vi "PH_Switch.calc State.vi"(0 "i ref in":refnum<vi>, 5 "error in (no error)":errorcluster) -> (14 "i ref out":refnum<vi>, 19 "error out":errorcluster)   [LabVIEW 2014, in "PH_Switch.lvlib"]
doc: "This VI calculates the device state and writes it in case of a change to own attributes and publishes it via DIM."
uses:
  PH_Switch.lvlib
  PH_StatusHandler/PH_StatusHandler.Status.ctl
  PH_StatusHandler/PH_StatusHandler.lvlib
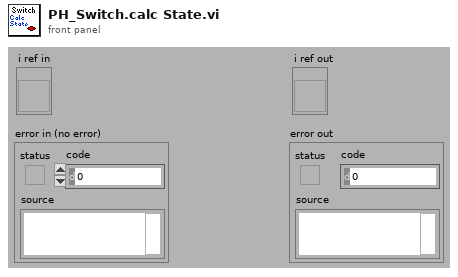
[diagram p1: front panel]
types:
  T1 = enum8{"Enabled", "Disabled", "Disabled and Grayed Out"}
  T2 = typedef "PH_StatusHandler.lvlib/PH_StatusHandler.Status.ctl" = i16
  T3 = typedef "PH_Switch.lvlib/PH_Switch.i attribute.ctl" = cluster{"GUI Refs":T4, "Status true":T2, "Status false":T2, "Status Switch State":T2, "remote controlled":bool, "Tagname":cluster{"Switch":string, "True":string, "False":string}, "Beckhoff Instance":string, "Caption":cluster{"True":string, "False":string}, "Default State":string}
  T4 = typedef "PH_Switch.lvlib/PH_Switch.GUI Refs.ctl" = cluster{"true":refnum<vi>, "false":refnum<vi>, "Switch_state":refnum<vi>, "GUI-Knob":refnum<vi>, "Delete":refnum<vi>, "Function Textfield":refnum<vi>}
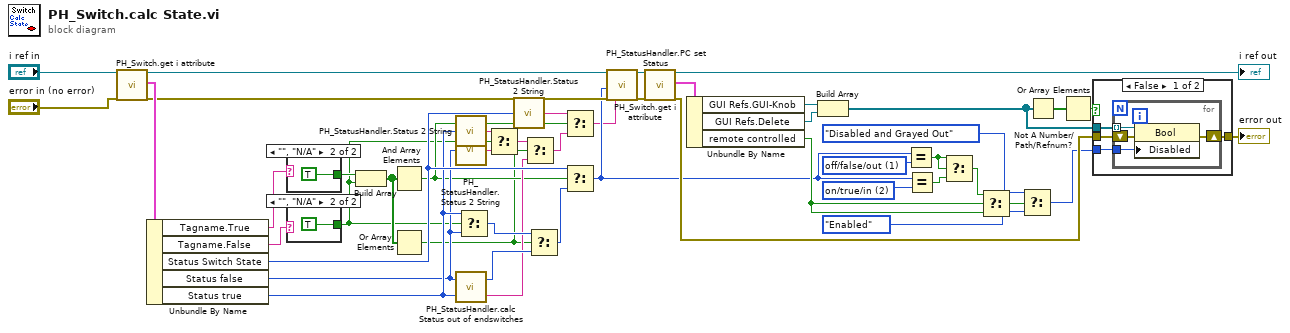
[diagram p0: block diagram]
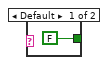
[diagram p3: hidden frame]
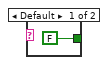
[diagram p4: hidden frame]
diagram:
  w23 = T2 2 items=["no info", "off/false/out", "on/true/in", "Failure", "Alarm", "Status 1", "Status 2", "Status 3"] ("Status")
  w27 = T2 1 items=["no info", "off/false/out", "on/true/in", "Failure", "Alarm", "Status 1", "Status 2", "Status 3"] ("Status")
  n1 = call "PH_Switch.get i attribute.vi"("i ref in"="i ref in", "error in (no error)"="error in (no error)") -> ("i ref out"=w19:refnum<vi>, "i attribute"=w40:T3, "error out"=w20:errorcluster)  [unwired: 15 in]
  n2 = Unbundle By Name(w40) -> ("Tagname.True"=w22:string, "Tagname.False"=w21:string, "Status Switch State"=w11:T2, "Status false"=w9:T2, "Status true"=w10:T2)
  n3 = case shown="\"\", \"N/A\"" w22 {
    tunnel: [FALSE TRUE] -> w41
    frame Default {
    }
    frame "", "N/A" {
    }
  }
  n4 = case shown="\"\", \"N/A\"" w21 {
    tunnel: [FALSE TRUE] -> w2
    frame Default {
    }
    frame "", "N/A" {
    }
  }
  n5 = Build Array(w41, w2) -> (w42:bool[])
  n6 = And Array Elements(Boolean array=w42) -> (logical AND=w4:bool)
  n7 = Or Array Elements(Boolean array=w42) -> (logical OR=w3:bool)
  n8 = call "PH_StatusHandler.Status 2 String.vi"("Status"=w10) -> ("Status as string"=w7:string)
  n9 = call "PH_StatusHandler.Status 2 String.vi"("Status"=w9) -> ("Status as string"=w6:string)
  n10 = call "PH_StatusHandler.calc Status out of endswitches.vi"("Status Input 2: \"True\""=w10, "Status Input 1: \"False\""=w9) -> ("Further Information"=w5:string, "Status Output"=w43:T2)
  n11 = Select(t=w10, s=w2, f=w9) -> (s? t:f=w45:T2)
  n12 = Select(t=w7, s=w2, f=w6) -> (s? t:f=w13:string)
  n13 = call "PH_StatusHandler.Status 2 String.vi"("Status"=w11) -> ("Status as string"=w8:string)
  n14 = Select(t=w13, s=w3, f=w5) -> (s? t:f=w12:string)
  n15 = Select(t=w45, s=w3, f=w43) -> (s? t:f=w44:T2)
  n16 = Select(t=w8, s=w4, f=w12) -> (s? t:f=w1:string)
  n17 = Select(t=w11, s=w4, f=w44) -> (s? t:f=w16:T2)
  n18 = call "PH_StatusHandler.PC set Status.vi"("i ref in"=w19, "Status"=w16, "error in (no error)"=w20, "Tip Strip"=w1) -> ("i ref out"=w18:refnum<vi>, "error out"=w17:errorcluster)  [unwired: 14 in]
  n19 = call "PH_Switch.get i attribute.vi"("i ref in"=w18, "error in (no error)"=w17) -> ("i ref out"=→"i ref out":refnum<vi>, "i attribute"=w39:T3, "error out"=w31:errorcluster)  [unwired: 15 in]
  n20 = Unbundle By Name(w39) -> ("GUI Refs.GUI-Knob"=w38:refnum<vi>, "GUI Refs.Delete"=w37:refnum<vi>, "remote controlled"=w29:bool)
  n21 = Build Array(w38, w37) -> (w36:refnum<vi>[])
  n22 = Equal?(x=w16, y=w27) -> (x = y?=w26:bool)
  n23 = Equal?(x=w16, y=w23) -> (x = y?=w24:bool)
  n24 = Select(t=w26, s=w26, f=w24) -> (s? t:f=w25:bool)
  n25 = Select(t=w25, s=w29, f=w29) -> (s? t:f=w28:bool)
  n26 = Select(t=T1."Disabled and Grayed Out" ("Disabled"), s=w28, f=T1."Enabled" ("Disabled")) -> (s? t:f=w30:T1)
  n27 = Not A Number/Path/Refnum?(number/path/refnum=w36) -> (NaN/Path/Refnum?=w35:bool[])
  n28 = Or Array Elements(Boolean array=w35) -> (logical OR=w34:bool)
  n29 = case shown="False" w34 {
    tunnel: w36 -> [w55 _]
    tunnel: w31 -> [w54 w60]
    tunnel: [w53 w60] -> w33
    tunnel: w30 -> [w52 _]
    frame False {
      n30 = for {
        tunnel: w55 -> [w59] mode=indexing
        tunnel: w52 -> [w56]
        shift-right: [w57] -> w53
        shift-left: w54 -> [w58]
        n31 = property class="Bool"(reference=w59, error in=w58, "Disabled"=w56) -> (error out=w57:errorcluster)  [unwired: 1 out]
      }
    }
    frame True {
    }
  }
  "error out" <- w33
